vi "your step name here Curve Name Replace.vi"(8 "Hardware in":string, 9 "Step Setup in":string, 10 "Setup in":T1={"No.VI"=0, "Category"="", "StepName"="", "Seq setup flattened"="", "Comment"="", "Steps config."=[], "Jump config"=[], "Start"=0.0, "Increment"=0.0, "Name"="Pa", "Unit"="Pa", "Y data"=1, "Y prefix"="", "Y dB ref"=1.0, "Y unit"="", "Repeat State Array"=[]} {"Repeat State Array"."Start" format="%#_5g"; "Y dB ref" format="%.1f"; "Y data" items=["dB", "Lin"]; "Start" format="%#_5g"}, 11 "Type In":string) -> (3 "Inserted Names Out":string[](array[string]))   [LabVIEW 2013]
uses:
  CRYCustom and Run Seq.llb/CRYStep.ctl
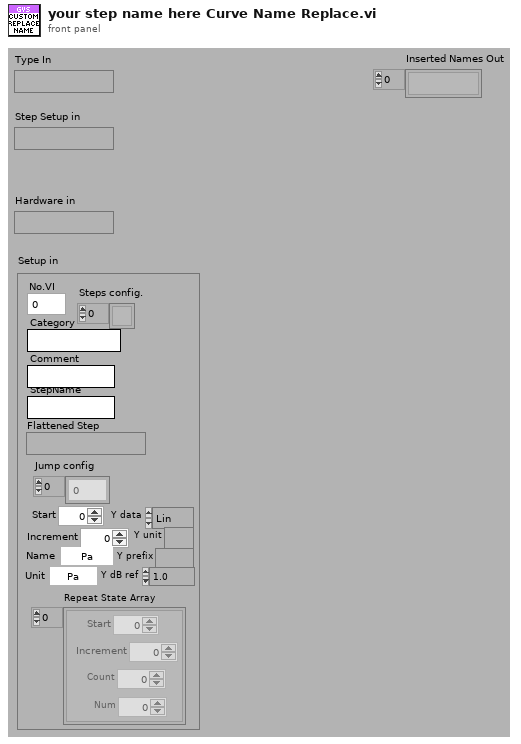
[diagram p1: front panel]
types:
  T1 = typedef "CRYStep.ctl" = cluster{"No.VI":i32, "Category":string, "StepName":string, "Seq setup flattened":string, "Comment":string, "Steps config.":bool[], "Jump config":i32[], "Start":dbl, "Increment":dbl, "Name":string, "Unit":string, "Y data":u16, "Y prefix":string, "Y dB ref":dbl, "Y unit":string, "Repeat State Array":cluster{"Start":dbl, "Increment":dbl, "Count":i32, "Num":i32}[]}
  T2 = cluster{"Parameter A":dbl, "Parameter B":dbl, "Parameter C":dbl}
  T3 = typedef "CRYCustom Cluster.ctl" = cluster{"Help":string, "Flatten Data":string}
  T4 = typedef "CRYData Cluster.ctl" = cluster{"Name":string, "Curve":cluster{"x":dbl, "y":dbl, "z":dbl}[], "X data":u16, "Y data":u16, "Z data":u16, "X axis":u16, "Y axis":u16, "Z axis":u16, "X unit":string, "Y unit":string, "Z unit":string, "X dB ref":dbl, "Y dB ref":dbl, "Z dB ref":dbl, "single val":bool, "protected":bool, "display X":bool, "display Y":bool, "display Z":bool, "Test Info":string, "Step No.":i32, "Plot Settings":cluster{"Color":u32, "Interpolation":u8, "Point Style":u8, "Line Style":u8, "Point Color":u32, "Line Width":u8, "Bar Plot Style":u8, "Fill To":i16}, "AutoProtect":bool}
  T5 = typedef "CRYWaveform Cluster.ctl" = cluster{"Waveform":cluster{"X0":dbl, "dX":dbl, "Y":sgl[]}, "X data":u16, "Y data":u16, "Y axis":u16, "X unit":string, "Y unit":string, "Y dB ref":dbl, "display Y":bool, "display X":bool, "Overload?":bool, "Test Info":string, "Step No.":i32, "Name":string, "protected":bool, "Sqc history":string[], "Signal Channel ID":i32, "Plot Settings":cluster{"Color":u32, "Interpolation":u8, "Point Style":u8, "Line Style":u8, "Point Color":u32, "Line Width":u8, "Bar Plot Style":u8, "Fill To":i16}, "AutoProtect":bool}
  T6 = typedef "CRYResult Cluster.ctl" = cluster{"Name":string, "Margin":dbl, "unit":string, "Verdict":bool, "Limit":string, "Max/Min":string, "protected":bool, "Step No.":i32, "Test Info":string, "AutoProtect":bool}
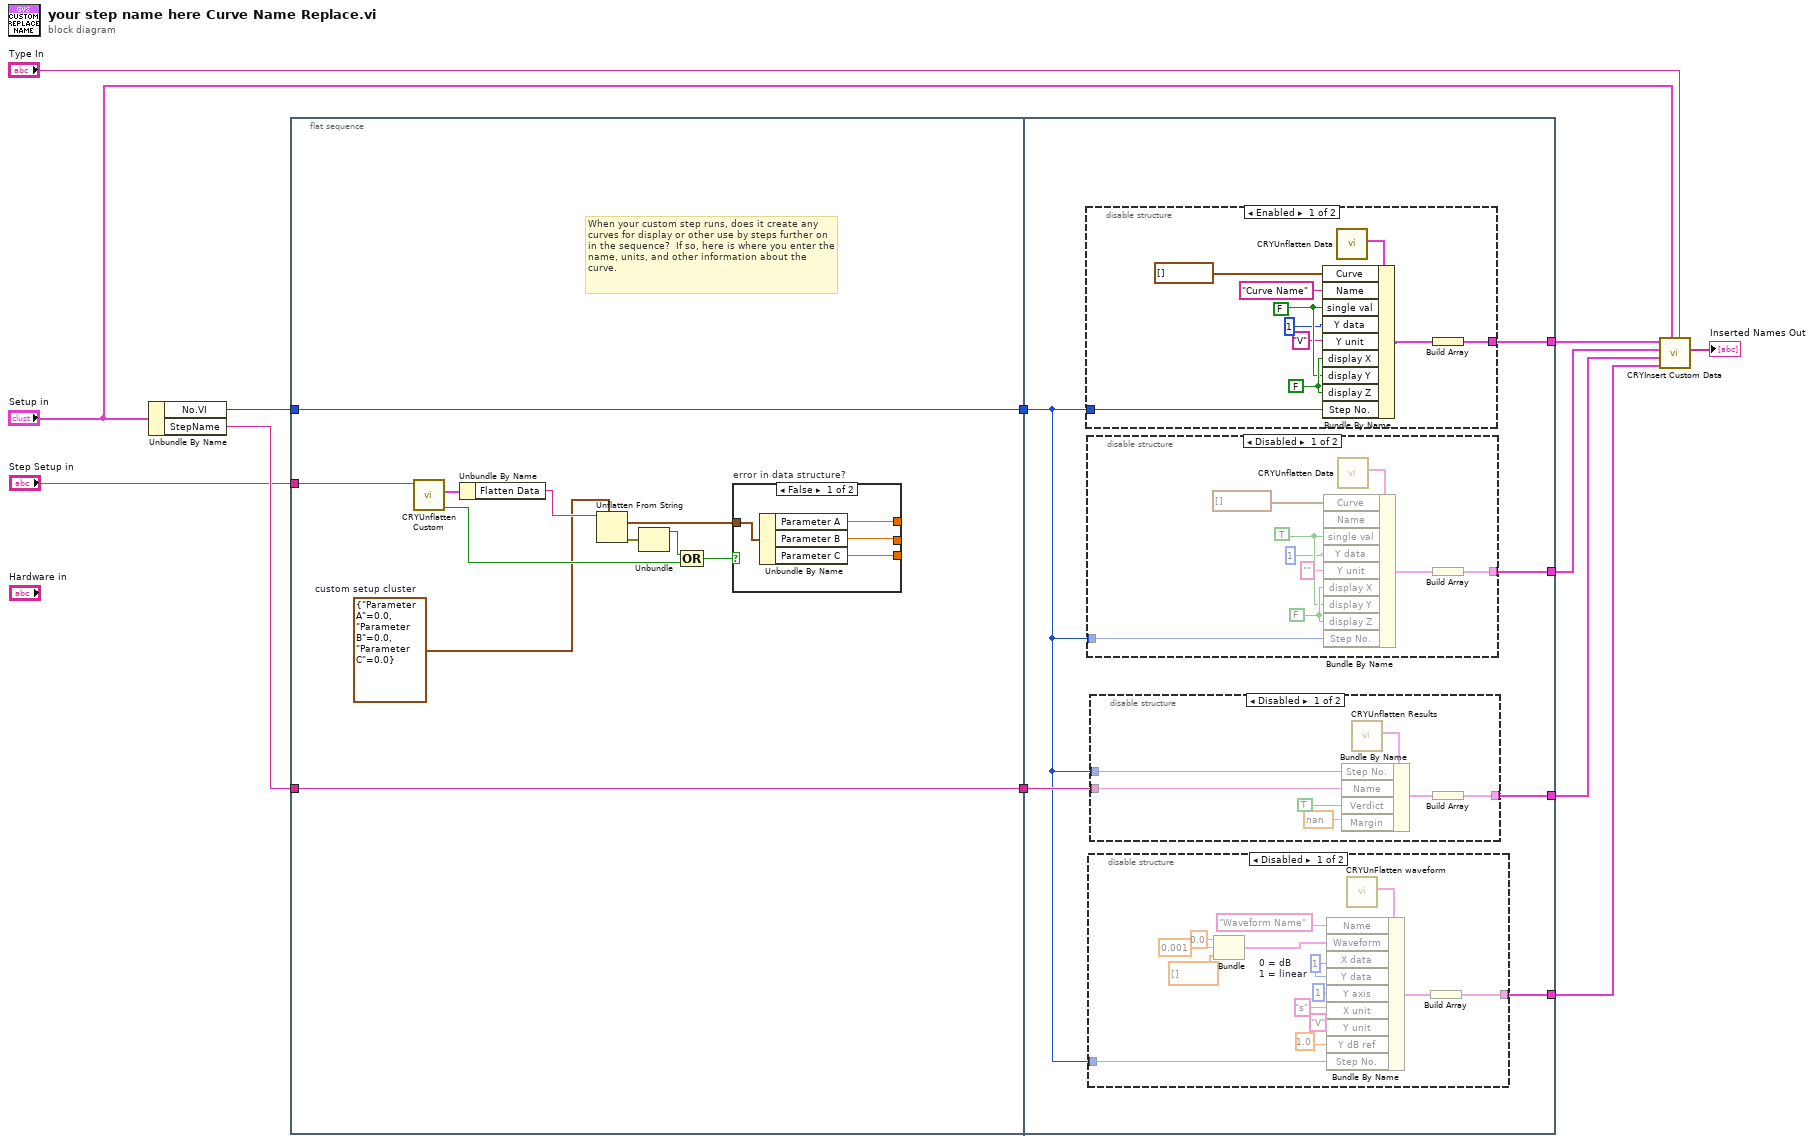
[diagram p0: block diagram]
diagram:
  n1 = Unbundle By Name("Setup in") -> ("No.VI"=w9:i32, "StepName"=w10:string)
  n2 = flat-sequence {
    tunnel: w9 -> [w22]
    tunnel: w10 -> [w23]
    tunnel: [w23] -> w4
    tunnel: [w22] -> w3
    tunnel: "Step Setup in" -> [w14]
    tunnel: [w31] -> w8
    tunnel: [w30] -> w6
    tunnel: [w29] -> w5
    tunnel: [w28] -> w7
    tunnel: w4 -> [w33]
    tunnel: w3 -> [w32]
    frame #0 {
      w13 = T2 {"Parameter A"=0.0, "Parameter B"=0.0, "Parameter C"=0.0}  # custom setup cluster
      # "When your custom step runs, does it create any curves for display or other use by steps further on in the sequence?  If so, here is where you enter the name, units, and other information about the curve."
      n3 = call "CRYUnflatten Custom.vi"("Unflatten Custom"=w14) -> ("Error?"=w15:bool, "Custom"=w17:T3)  [unwired: 8 in, 1 out]
      n4 = Unbundle By Name(w17) -> ("Flatten Data"=w16:string)
      n5 = Unflatten From String(type=w13, binary string=w16) -> (value=w20:T2, error out=w21:errorcluster)  [unwired: 1 in, 3 out]
      n6 = Unbundle(w21) -> ("status"=w18:bool)  [unwired: 2 out]
      n7 = Compound Arithmetic op=OR(w18, w15) -> (w19:bool)
      n8 = case "error in data structure?" shown="False" w19 {
        tunnel: w20 -> [w27 _]
        tunnel: [w26 _] -> _
        tunnel: [w25 _] -> _
        tunnel: [w24 _] -> _
        frame False {
          n9 = Unbundle By Name(w27) -> ("Parameter A"=w26:dbl, "Parameter B"=w25:dbl, "Parameter C"=w24:dbl)
        }
        frame True {
        }
      }
    }
    frame #1 {
      n10 = disable-structure shown="Enabled" {
        disable-tunnel: w32 -> [w39 _]
        disable-tunnel: [w34 _] -> w31
        frame Enabled {
          w42 = FALSE
          w41 = FALSE
          n11 = call "CRYUnflatten Data.vi"() -> ("Datum"=w43:T4)  [unwired: 9 in, 2 out]
          n12 = Bundle By Name(cluster=w43, "Curve"=cluster{"x":dbl, "y":dbl, "z":dbl}[] [] ("appended array"), "Name"="Curve Name", "single val"=w41, "Y data"=u16 1, "Y unit"="V", "display X"=w42, "display Y"=w41, "display Z"=w42, "Step No."=w39) -> (w35:T4)
          n13 = Build Array(w35) -> (w34:T4[])
        }
        frame Disabled {
        }
      }
      n14 = disable-structure shown="Disabled" {
        disable-tunnel: w32 -> [w48 _]
        disable-tunnel: [w46 _] -> w28
        frame Disabled {
          w51 = FALSE
          w50 = TRUE
          n15 = call "CRYUnflatten Data.vi"() -> ("Datum"=w52:T4)  [unwired: 9 in, 2 out]
          n16 = Bundle By Name(cluster=w52, "Curve"=cluster{"x":dbl, "y":dbl, "z":dbl}[] [] ("appended array"), "single val"=w50, "Y data"=u16 1, "Y unit"="", "display X"=w51, "display Y"=w50, "display Z"=w51, "Step No."=w48) -> (w47:T4)  [unwired: 1 in]
          n17 = Build Array(w47) -> (w46:T4[])
        }
        frame Enabled {
        }
      }
      n18 = disable-structure shown="Disabled" {
        disable-tunnel: [w61 _] -> w29
        disable-tunnel: w32 -> [w60 _]
        frame Disabled {
          w66 = u16 1  # 0 = dB 1 = linear
          n19 = Bundle ("Actual waveform data bundle.\nX0\ndX\n[Y] array")(0.0, 0.001, dbl[] []) -> (w70:cluster{dbl, dbl, dbl[]})  [unwired: 1 out]
          n20 = call "CRYUnFlatten waveform.vi"() -> ("Waveform Cluster"=w71:T5)  [unwired: 9 in, 2 out]
          n21 = Bundle By Name(cluster=w71, "Name"="Waveform Name" ("Bundle Element"), "Waveform"=w70, "X data"=w66, "Y data"=w66, "Y axis"=u16 1, "X unit"="s", "Y unit"="V", "Y dB ref"=1.0, "Step No."=w60) -> (w72:T5)
          n22 = Build Array(w72) -> (w61:T5[])
        }
        frame Enabled {
        }
      }
      n23 = disable-structure shown="Disabled" {
        disable-tunnel: w32 -> [w55 _]
        disable-tunnel: w33 -> [w54 _]
        disable-tunnel: [w53 _] -> w30
        frame Disabled {
          n24 = call "CRYUnflatten Results.vi"() -> ("Result"=w56:T6)  [unwired: 9 in, 2 out]
          n25 = Bundle By Name(cluster=w56, "Step No."=w55, "Name"=w54, "Verdict"=TRUE, "Margin"=nan) -> (w58:T6)
          n26 = Build Array(w58) -> (w53:T6[])
        }
        frame Enabled {
        }
      }
    }
  }
  n27 = call "CRYInsert Custom Data.vi"("sAction"="Type In", "Setup in"="Setup in", "Wave"=w5, "Results"=w6, "Values"=w7, "Curves"=w8) -> ("Inserted Names Out"=→"Inserted Names Out":string[])  [unwired: 4 in, 1 out]
